vi "Log Build.vi"() -> ()   [LabVIEW 2016]
panel:
  out "element":string
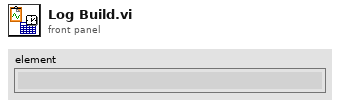
[diagram p1: front panel]
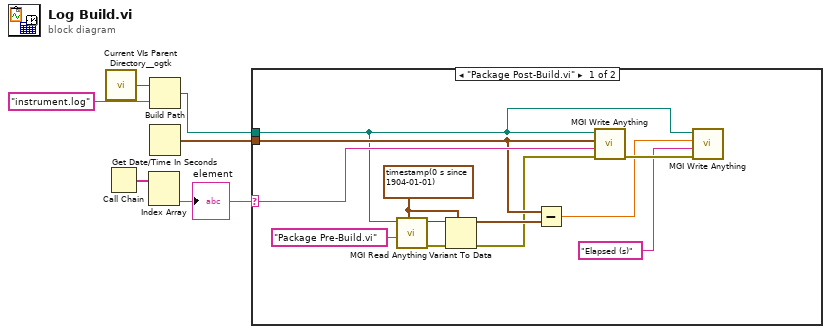
[diagram p0: block diagram]
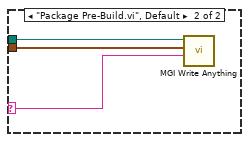
[diagram p2: hidden frame]
diagram:
  n1 = call <userlib>:"Current VIs Parent Directory__ogtk.vi"() -> ("Parent Directory (+ Relative)"=w4:path)  [unwired: 5 in]
  n2 = Call Chain() -> (call chain=w6:string[])
  n3 = Index Array(array=w6) -> (element #2=w1:string)  [unwired: 2 in, 1 out]
  "element" <- w1
  n4 = Build Path(base path=w4, name or relative path="instrument.log") -> (appended path=w3:path)
  n5 = Get Date/Time In Seconds() -> (seconds since 1Jan1904=w2:timestamp)
  n6 = case shown="\"Package Post-Build.vi\"" w1 {
    selector: w1 -> [w18 w19]
    tunnel: w3 -> [w9 w21]
    tunnel: w2 -> [w12 w20]
    frame "Package Post-Build.vi" {
      w15 = timestamp(0 s since 1904-01-01) ("Time Stamp")
      n7 = call <userlib>:"MGI Read Anything.vi"("Type of Anything"=w15, "Section Name (Name of \"Type of Anything\")"="Package Pre-Build.vi" ("Section Name (Name of \"Type of Anything\")"), "Path (dialog)"=w9) -> ("Error Out"=w17:errorcluster, "Anything"=w16:variant)  [unwired: 5 in, 2 out]
      n8 = Variant To Data(error in=w17, type=w15, Variant=w16) -> (data=w13:timestamp, error out=w10:errorcluster)
      n9 = Subtract(x=w12, y=w13) -> (x-y=w8:dbl)
      n10 = call <userlib>:"MGI Write Anything.vi"("Error In"=w10, "Section Name (Name of \"Anything\")"=w18, "Anything"=w12, "Path (dialog)"=w9) -> ("Error Out"=w11:errorcluster)  [unwired: 5 in, 2 out]
      n11 = call <userlib>:"MGI Write Anything.vi"("Error In"=w11, "Section Name (Name of \"Anything\")"="Elapsed (s)" ("Section Name (Name of \"Anything\")"), "Anything"=w8, "Path (dialog)"=w9) -> ()  [unwired: 5 in, 3 out]
    }
    frame "Package Pre-Build.vi", Default {
      n12 = call <userlib>:"MGI Write Anything.vi"("Section Name (Name of \"Anything\")"=w19, "Anything"=w20, "Path (dialog)"=w21) -> ()  [unwired: 6 in, 3 out]
    }
  }
